vi "Zero Channel.vi"(8 "error in (no error)":errorcluster, 9 "Dev to Zero":i32=1, 10 "Channel Array":refnum<k21>[](array[refnum]), 11 "Refnum":refnum<vi>) -> (0 "error out":errorcluster, 3 "Zero Values":dbl[](array[numeric]))   [LabVIEW 2017]
uses:
  <vilib>/DAQmx/read.llb/DAQmx Read (Analog 2D DBL NChan NSamp).vi
  <vilib>/DAQmx/miscellaneous.llb/DAQmx Fill In Error Info.vi
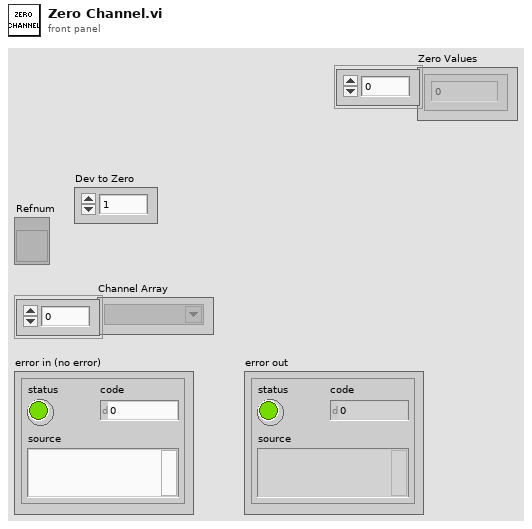
[diagram p1: front panel]
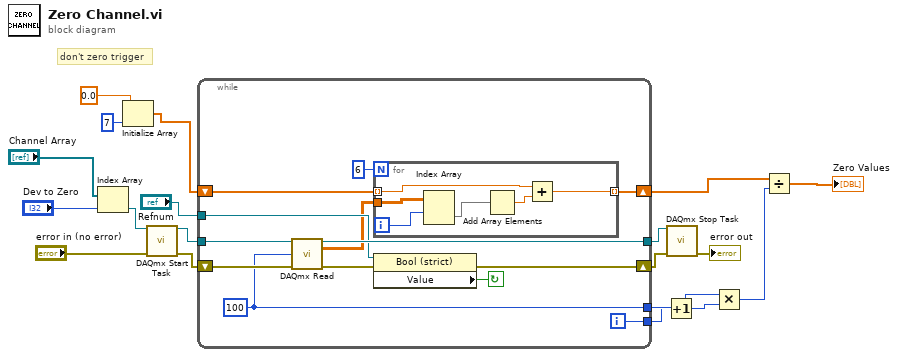
[diagram p0: block diagram]
diagram:
  # "don't zero trigger"
  n1 = Index Array(array="Channel Array", index="Dev to Zero") -> (element=w7:refnum<k21>)
  n2 = Initialize Array(0.0 ("element"), 7 ("dimension size")) -> (w1:dbl[])
  n3 = call <vilib>:"DAQmx Start Task.vi"("task/channels in"=w7, "error in"="error in (no error)") -> ("task out"=w9:refnum<k21>, "error out"=w10:errorcluster)  [unwired: 12 in]
  n4 = while {
    tunnel: w9 -> [w32]
    tunnel: [w30] -> w16
    tunnel: [w29] -> w13
    shift-right: [w25] -> w11
    shift-left: w10 -> [w31]
    tunnel: [w28] -> w17
    tunnel: "Refnum" -> [w27]
    shift-right: [w22] -> w5
    shift-left: w1 -> [w21]
    i -> [w30]
    stop <- w26 continue-if-true
    w28 = 100 ("number of samples per channel")
    n5 = call-poly <vilib>:"DAQmx Read.vi"("task/channels in"=w32, "number of samples per channel"=w28, "error in"=w31) -> ("task out"=w29:refnum<k21>, "data"=w23:dbl[][], "error out"=w24:errorcluster)  [unwired: 10 in]
    n6 = for {
      N: 6 -> [_]
      tunnel: w23 -> [w35]
      tunnel: [w37] -> w22 mode=indexing
      tunnel: w21 -> [w33] mode=indexing
      i -> [w36]
      n7 = Index Array(array=w35, index (row)=w36) -> (element=w34:dbl[])  [unwired: 1 in]
      n8 = Add Array Elements(numeric array=w34) -> (sum=w38:dbl)
      n9 = Add(x=w33, y=w38) -> (x+y=w37:dbl)
    }
    n10 = property class="Bool (strict)"(reference=w27, error in=w24) -> (error out=w25:errorcluster, "Value"=w26:bool)  [unwired: 1 out]
  }
  n11 = Increment(x=w16) -> (x+1=w18:i32)
  n12 = call <vilib>:"DAQmx Stop Task.vi"("task/channels in"=w13, "error in"=w11) -> ("error out"=→"error out":errorcluster)  [unwired: 12 in, 1 out]
  n13 = Multiply(x=w17, y=w18) -> (x*y=w15:i32)
  n14 = Divide(x=w5, y=w15) -> (x/y=→"Zero Values":dbl[])
